vi "Eurotherm - Calculate Sensor Reading.vi"(0 "Eurotherm Setup In":T1={"Communication"={"Com Port"=1, "Address"=1, "Baud Rate"=9600}, "Name"="", "Enable"=FALSE, "Max Set Point"=0.0, "Min Set Point"=0.0, "Units"="", "Graph Data"=0, "Sensor type"=enum."RhFe", "Calibration File Path"=path "", "Conversion Type"=enum."Linear"} {"Min Set Point" format="%.3f"; "Max Set Point" format="%.3f"; "Communication"."Baud Rate" items=["300"=300, "600"=600, "1200"=1200, "2400"=2400, "4800"=4800, "9600 (default)"=9600, "19200"=19200, "38400"=38400, "57600"=57600, "76800"=76800, "115200"=115200, "230400"=230400]; "Communication"."Com Port" min=1 max=255; "Communication"."Address" min=1 max=99}, 7 "Measured Value":dbl format="%.3f", 11 "error in (no error)":errorcluster) -> (4 "Eurotherm Setup Out":T1={"Communication"={"Com Port"=1, "Address"=1, "Baud Rate"=9600}, "Name"="", "Enable"=FALSE, "Max Set Point"=0.0, "Min Set Point"=0.0, "Units"="", "Graph Data"=0, "Sensor type"=enum."RhFe", "Calibration File Path"=path "", "Conversion Type"=enum."Linear"} {"Min Set Point" format="%.3f"; "Max Set Point" format="%.3f"; "Communication"."Baud Rate" items=["300"=300, "600"=600, "1200"=1200, "2400"=2400, "4800"=4800, "9600 (default)"=9600, "19200"=19200, "38400"=38400, "57600"=57600, "76800"=76800, "115200"=115200, "230400"=230400]; "Communication"."Com Port" min=1 max=255; "Communication"."Address" min=1 max=99}, 8 "Converted Value":dbl format="%.3f", 15 "error out":errorcluster)   [LabVIEW 2011]
uses:
  Eurotherm - Controls/Eurotherm - Setup.ctl
  Eurotherm - Controls/Eurotherm - Communication.ctl
  Common/Utilities/Controls - Com Ports/Com Port - Numeric.ctl
  Eurotherm - Controls/Eurotherm - Address.ctl
  Common/Utilities/Controls - Com Ports/Com Port - Baud Rate.ctl
  Common/Utilities - System/Sensors/Sensors - Controls/Sensors - Temperature Sensor Type.ctl
  Common/Utilities - System/Sensors/Sensors - Controls/Sensors - Conversion Type.ctl
  Common/Utilities - System/Sensors/Sensors - Controls/Sensors - Translation Type.ctl
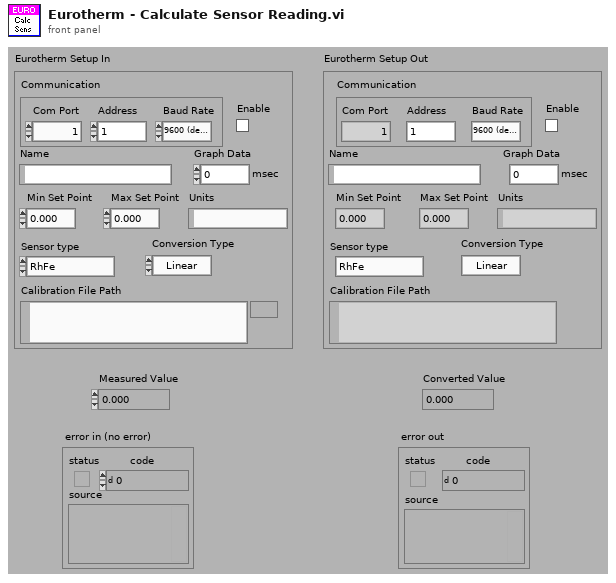
[diagram p1: front panel]
types:
  T1 = typedef "Eurotherm - Setup.ctl" = cluster{"Communication":T2, "Name":string, "Enable":bool, "Max Set Point":dbl, "Min Set Point":dbl, "Units":string, "Graph Data":u32, "Sensor type":T6, "Calibration File Path":path, "Conversion Type":T7}
  T2 = typedef "Eurotherm - Communication.ctl" = cluster{"Com Port":T3, "Address":T4, "Baud Rate":T5}
  T3 = typedef "Com Port - Numeric.ctl" = i32
  T4 = typedef "Eurotherm - Address.ctl" = u8
  T5 = typedef "Com Port - Baud Rate.ctl" = u32
  T6 = typedef "Sensors - Temperature Sensor Type.ctl" = enum16{"RhFe", "Pt", "K type thermocouple", "W5 type thermocouple", "No Conversion"}
  T7 = typedef "Sensors - Conversion Type.ctl" = enum16{"Linear", "Spline"}
  T8 = typedef "Sensors - Translation Type.ctl" = enum16{"K/C", "mV"}
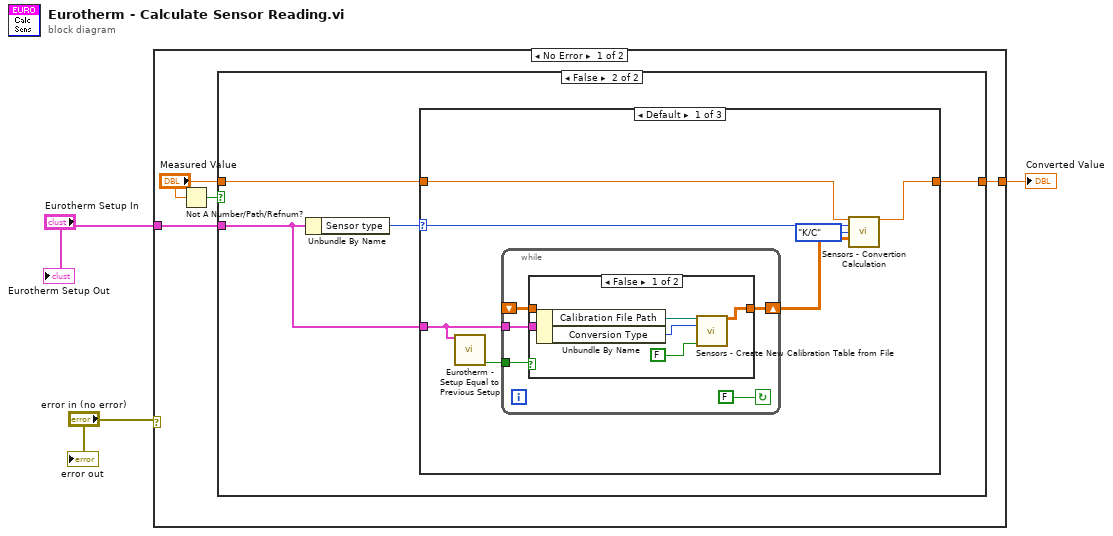
[diagram p0: block diagram]
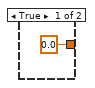
[diagram p2: hidden frame]
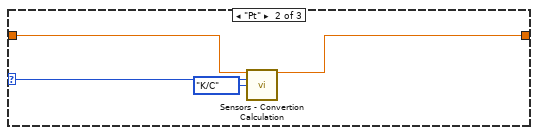
[diagram p4: hidden frame]
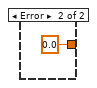
[diagram p6: hidden frame]
diagram:
  n1 = case shown="No Error" "error in (no error)" {
    tunnel: [w7 0.0] -> w3
    tunnel: "Eurotherm Setup In" -> [w4 _]
    frame No Error {
      n2 = Not A Number/Path/Refnum?(number/path/refnum="Measured Value") -> (NaN/Path/Refnum?=w5:bool)
      n3 = case shown="False" w5 {
        tunnel: "Measured Value" -> [_ w11]
        tunnel: [0.0 w10] -> w7
        tunnel: w4 -> [_ w9]
        frame True {
        }
        frame False {
          n4 = Unbundle By Name(w9) -> ("Sensor type"=w12:T6)
          n5 = case shown="Default" w12 {
            selector: w12 -> [w17 w34 _]
            tunnel: w11 -> [w19 w32 w35]
            tunnel: [w18 w31 w35] -> w10
            tunnel: w9 -> [w15 _ _]
            frame Default {
              n6 = call "Eurotherm - Setup Equal to Previous Setup.vi"("Value In"=w15) -> ("Equal to previous value"=w14:bool)  [unwired: 13 in, 1 out]
              n7 = while {
                tunnel: w15 -> [w24]
                shift-right: [w23] -> w13
                shift-left: _ -> [w21]
                tunnel: w14 -> [w22]
                stop <- FALSE continue-if-true
                n8 = case shown="False" w22 {
                  tunnel: w24 -> [w29 _]
                  tunnel: [w25 w30] -> w23
                  tunnel: w21 -> [_ w30]
                  frame False {
                    n9 = Unbundle By Name(w29) -> ("Calibration File Path"=w28:path, "Conversion Type"=w27:T7)
                    n10 = call "Sensors - Create New Calibration Table from File.vi"("Calibration Data File"=w28, "Conversion Type"=w27, "Write table to file"=FALSE) -> ("Output Table"=w25:dbl[][])  [unwired: 12 in]
                  }
                  frame True {
                  }
                }
              }
              n11 = call "Sensors - Convertion Calculation.vi"("Input Value"=w19, "Sensor type"=w17, "Translate To"=Sensors_-_Translation_Type."K/C", "Input Table"=w13) -> ("Output Value"=w18:dbl)  [unwired: 10 in, 1 out]
            }
            frame "Pt" {
              n12 = call "Sensors - Convertion Calculation.vi"("Input Value"=w32, "Sensor type"=w34, "Translate To"=Sensors_-_Translation_Type."K/C") -> ("Output Value"=w31:dbl)  [unwired: 11 in, 1 out]
            }
            frame "No Conversion" {
            }
          }
        }
      }
    }
    frame Error {
    }
  }
  "Converted Value" <- w3
  "error out" <- "error in (no error)"
  "Eurotherm Setup Out" <- "Eurotherm Setup In"
